vi "save_bin_trace.vi"(8 "Decimate":i32=1, 10 "File path":path) -> ()   [LabVIEW 2013]
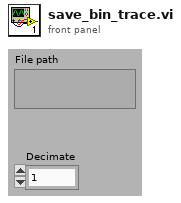
[diagram p1: front panel]
types:
  T1 = enum16{"big-endian, network order", "native, host order", "little-endian"}
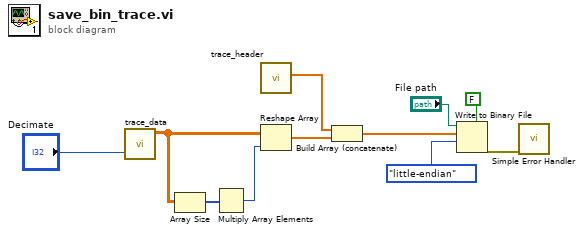
[diagram p0: block diagram]
diagram:
  n1 = call "trace_data.vi"("Decimate"="Decimate") -> ("Decimated trace"=w5:sgl[][][])  [unwired: 8 in, 2 out]
  n2 = Array Size(array=w5) -> (size(s)=w4:i32[])
  n3 = Multiply Array Elements(1:w4) -> (0:w3:i32)
  n4 = call "trace_header.vi"() -> ("Header"=w1:sgl[])  [unwired: 11 in]
  n5 = Reshape Array(w5, w3) -> (w2:sgl[])
  n6 = Build Array (concatenate)(w1, w2) -> (w6:sgl[])
  n7 = Write to Binary File(file (use dialog)="File path", data=w6, 5:FALSE ("prepend array or string size? (T)"), 9:T1."little-endian" ("byte order (0:big-endian, network order)")) -> (error out=w8:errorcluster)  [unwired: 1 in, 3 out]
  n8 = call <vilib>:"Simple Error Handler.vi"("error in (no error)"=w8) -> ()  [unwired: 1 in, 8 out]
